vi "List columns.vi"(8 "error in (no error)":errorcluster, 9 "显示关键参数":bool, 10 "table":string, 11 "database":string="database1.mdb") -> (0 "error out":errorcluster, 3 "columns":string[](array[string]))   [LabVIEW 2016, in "数据查询.lvlib"]
uses:
  <vilib>/addons/database/Connection.llb/DB Tools Open Connec (String).vi
  <userlib>/_LVST/sqlite_api/Core/Tables/SQLite_List Columns.vi
  <userlib>/_OpenG.lib/array/array.llb/Filter 1D Array (String)__ogtk.vi
  <vilib>/addons/database/NI_Database_API.lvlib
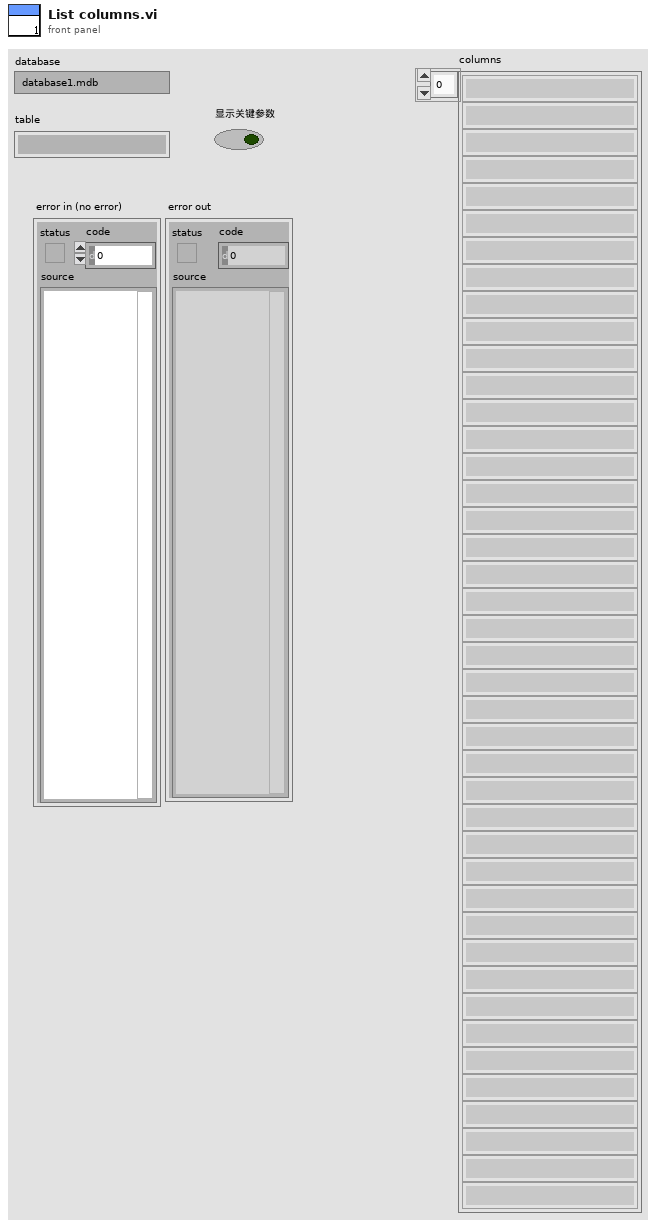
[diagram p1: front panel]
types:
  T1 = typedef "数据库类型.ctl" = enum16{"Access", "SQLite"}
  T2 = typedef "NI_Database_API.lvlib/Conn ObjectReference.ctl" = refnum<k1>
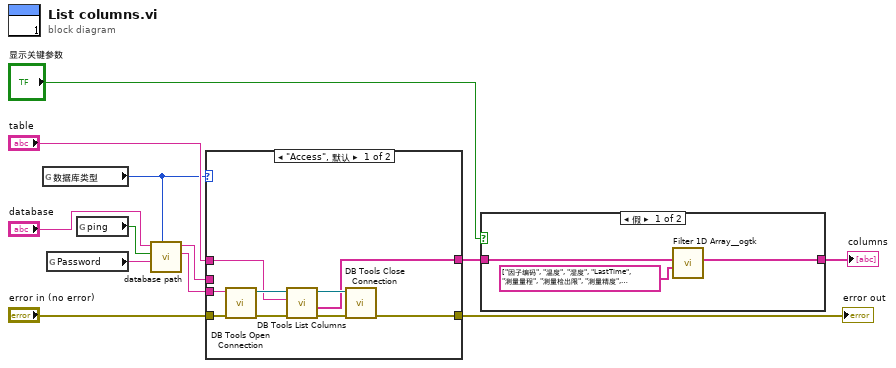
[diagram p0: block diagram]
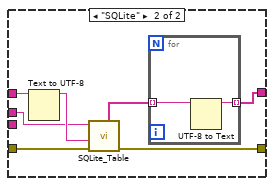
[diagram p3: hidden frame]
diagram:
  n1 = global read "全局变量.vi" "数据库类型"() -> (w7:T1)
  n2 = global read "全局变量.vi" "Password"() -> (w1:string)
  n3 = global read "全局变量.vi" "ping"() -> (w6:bool)
  n4 = call "database path.vi"("数据库类型"=w7, "Password"=w1, "ping"=w6, "database"="database") -> ("Connection information"=w2:string, "Path out"=w8:string)  [unwired: 6 in]
  n5 = case shown="\"Access\", 默认" w7 {
    tunnel: "table" -> [w17 w24]
    tunnel: "error in (no error)" -> [w16 w27]
    tunnel: [w15 w28] -> w10
    tunnel: [w14 w25] -> w4
    tunnel: w8 -> [_ w22]
    tunnel: w2 -> [w13 _]
    frame "Access", Default {
      n6 = call-poly <vilib>:"DB Tools Open Connection.vi"("error in (no error)"=w16, "connection information"=w13) -> ("error out"=w19:errorcluster, "connection reference"=w21:T2)  [unwired: 6 in]
      n7 = call <vilib>:"DB Tools List Columns.vi"("error in (no error)"=w19, "table"=w17, "connection reference"=w21) -> ("error out"=w18:errorcluster, "columns"=w14:string[], "connection reference out"=w20:T2)  [unwired: 1 in, 1 out]
      n8 = call <vilib>:"DB Tools Close Connection.vi"("error in (no error)"=w18, "connection reference"=w20) -> ("error out"=w15:errorcluster)  [unwired: 5 in]
    }
    frame "SQLite" {
      n9 = Text to UTF-8(11:w24) -> (3:w23:string)  [unwired: 2 in, 1 out]
      n10 = call-poly <userlib>:"SQLite_Table.vi"("DB Path"=w22, "Table Name"=w23, "error in (no error)"=w27) -> ("Columns"=w26:string[], "error out"=w28:errorcluster)  [unwired: 4 in, 2 out]
      n11 = for {
        tunnel: w26 -> [w30] mode=indexing
        tunnel: [w29] -> w25 mode=indexing
        n12 = UTF-8 to Text(11:w30) -> (3:w29:string)  [unwired: 2 in, 1 out]
      }
    }
  }
  "error out" <- w10
  n13 = case shown="假" "显示关键参数" {
    tunnel: w4 -> [w33 w34]
    tunnel: [w31 w34] -> w3
    frame False {
      n14 = call-poly <userlib>:"Filter 1D Array__ogtk.vi"("items to filter"=string[] ["因子编码", "温度", "湿度", "LastTime", "测量量程", "测量检出限", "测量精度", "测量间隔", "消解温度", "消解时长", "三项式系数", "二次多项式系数", "曲线斜率", "曲线截距", "线性相关系数", "空白校准时间", "标样校准时间", "测量信号值", "稀释倍数", "空白标定系数", "量程系数", "X1"] ("columns"), "array"=w33) -> ("filtered array"=w31:string[])  [unwired: 4 in, 1 out]
    }
    frame True {
    }
  }
  "columns" <- w3
